vi "checkIfControlInOldLibrary.vi"(8 "error in (no error)":errorcluster, 10 "Ctl Refnum":refnum<vi>, 11 "VI in":refnum<class "VI.lvclass">) -> (0 "error out":errorcluster, 1 "VI Reference":refnum<vi>, 2 "isMemberOfOldLibrary":bool, 3 "VI out":refnum<class "VI.lvclass">)   [LabVIEW 2016, in "VI.lvclass"]
uses:
  VI.lvclass
  C:/LSST_TS/SystemSW/ct_tools/ProjectItem/ProjectItem.lvclass
  ProjectItem/ProjectItem.lvclass/ProjectItem.ctl
  ProjectItem/ProjectItem.lvclass
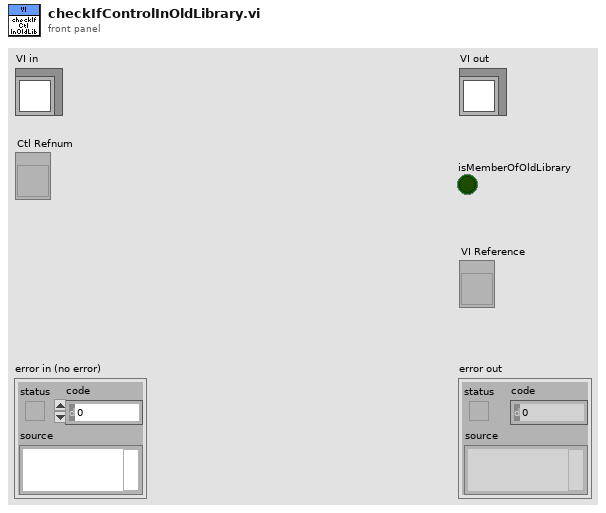
[diagram p1: front panel]
types:
  T1 = cluster{"OldLibrary":string, "NewLibrary":string}
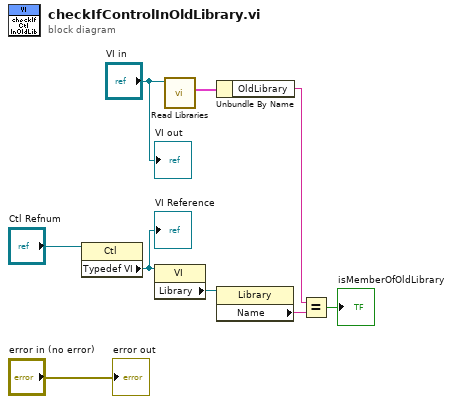
[diagram p0: block diagram]
diagram:
  n1 = property class="Ctl"(reference="Ctl Refnum") -> ("Typedef VI"=w2:refnum<vi>)  [unwired: 1 in, 2 out]
  "VI Reference" <- w2
  n2 = property class="VI"(reference=w2) -> ("Library"=w6:refnum<vi>)  [unwired: 1 in, 2 out]
  n3 = call "Read Libraries.vi"("ProjectItem in"="VI in") -> ("Libraries"=w7:T1)  [unwired: 9 in, 1 out]
  n4 = Unbundle By Name(w7) -> ("OldLibrary"=w5:string)
  n5 = property class="Library"(reference=w6) -> ("Name"=w4:string)  [unwired: 1 in, 2 out]
  n6 = Equal?(x=w5, y=w4) -> (x = y?=→"isMemberOfOldLibrary":bool)
  "error out" <- "error in (no error)"
  "VI out" <- "VI in"
